vi "merge segmented areas.vi"(6 "iterations (1)":i32, 9 "mergin array":i32[](array[numeric]), 10 "Array":u8[][](array[numeric]), 11 "Array 2":u8[][](array[numeric])) -> (0 "error out":errorcluster, 2 "Array out":u8[][](array[numeric]))   [LabVIEW 2018]
uses:
  <vilib>/vision/NI_Vision_Development_Module.lvlib
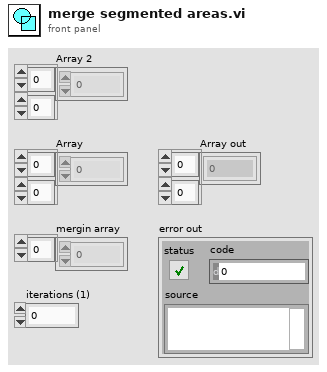
[diagram p1: front panel]
types:
  T1 = enum32{"AutoM", "Close", "Dilate", "Erode", "Gradient", "Gradient out", "Gradient in", "Hit miss", "Open", "PClose", "POpen", "Thick", "Thin"}
  T2 = typedef "Image Type" = u32
  T3 = typedef "IMAQ Image.ctl" = refnum<image>
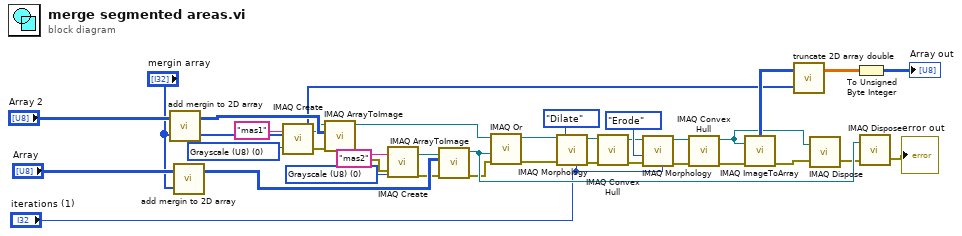
[diagram p0: block diagram]
diagram:
  w7 = T2 0 items=["Grayscale (U8)", "Grayscale (I16)", "Grayscale (SGL)", "Complex (CSG)", "RGB (U32)", "HSL (U32)", "RGB (U64)", "Grayscale (U16)"] ("Image Type")
  w11 = T2 0 items=["Grayscale (U8)", "Grayscale (I16)", "Grayscale (SGL)", "Complex (CSG)", "RGB (U32)", "HSL (U32)", "RGB (U64)", "Grayscale (U16)"] ("Image Type")
  n1 = call "add mergin to 2D array.vi"("mergin array"="mergin array", "Array in"="Array 2") -> ("Array out"=w30:u8[][])  [unwired: 1 in]
  n2 = call "add mergin to 2D array.vi"("mergin array"="mergin array", "Array in"="Array") -> ("Array out"=w31:u8[][])  [unwired: 1 in]
  n3 = call "IMAQ Create"("Image Name"="mas1", "Image Type"=w11) -> ("New Image"=w16:T3, "error out"=w13:errorcluster)  [unwired: 3 in]
  n4 = call "IMAQ ArrayToImage"("error in (no error)"=w13, "Image Pixels (U8)"=w30, "Image"=w16) -> ("error out"=w8:errorcluster, "Image Out"=w18:T3)  [unwired: 7 in]
  n5 = call "IMAQ Create"("Image Name"="mas2", "Image Type"=w7, "error in (no error)"=w8) -> ("New Image"=w15:T3, "error out"=w12:errorcluster)  [unwired: 2 in]
  n6 = call "IMAQ ArrayToImage"("error in (no error)"=w12, "Image Pixels (U8)"=w31, "Image"=w15) -> ("error out"=w19:errorcluster, "Image Out"=w28:T3)  [unwired: 7 in]
  n7 = call "IMAQ Or"("error in (no error)"=w19, "Image Src B"=w28, "Image Src A"=w18) -> ("error out"=w22:errorcluster, "Image Dst Out"=w20:T3)  [unwired: 7 in]
  n8 = call "IMAQ Morphology"("Number of iterations (1)"="iterations (1)", "error in (no error)"=w22, "Operation"=T1."Dilate", "Image Src"=w20) -> ("error out"=w23:errorcluster, "Image Dst Out"=w26:T3)  [unwired: 6 in]
  n9 = call "IMAQ Convex Hull"("error in (no error)"=w23, "Image Src"=w26) -> ("error out"=w24:errorcluster, "Image Dst Out"=w25:T3)  [unwired: 8 in]
  n10 = call "IMAQ Morphology"("Number of iterations (1)"="iterations (1)", "error in (no error)"=w24, "Operation"=T1."Erode", "Image Src"=w25) -> ("error out"=w33:errorcluster, "Image Dst Out"=w32:T3)  [unwired: 6 in]
  n11 = call "IMAQ Convex Hull"("error in (no error)"=w33, "Image Src"=w32) -> ("error out"=w34:errorcluster, "Image Dst Out"=w4:T3)  [unwired: 8 in]
  n12 = call "IMAQ ImageToArray"("error in (no error)"=w34, "Image"=w4) -> ("error out"=w3:errorcluster, "Image Pixels (U8)"=w35:u8[][])  [unwired: 2 in, 3 out]
  n13 = call "truncate 2D array double.vi"("b-t-l-r"="mergin array", "Array in"=w35) -> ("Array out"=w36:dbl[][])  [unwired: 1 in]
  n14 = call "IMAQ Dispose"("Image"=w4, "error in (no error)"=w3) -> ("error out"=w10:errorcluster)  [unwired: 4 in]
  n15 = To Unsigned Byte Integer(number=w36) -> (unsigned 8bit integer=→"Array out":u8[][])
  n16 = call "IMAQ Dispose"("Image"=w28, "error in (no error)"=w10) -> ("error out"=→"error out":errorcluster)  [unwired: 4 in]
